vi "Main.vi"() -> (0 "error out":errorcluster)   [LabVIEW 2010, in "Sound Demo.lvclass"]
doc: "This is the top-level VI that starts the Sound Player Demo application."
uses:
  Sound Demo.lvclass
  Application/Application.lvclass
panel:
  # "This is the top-level VI of the \nSound Player Demo project."
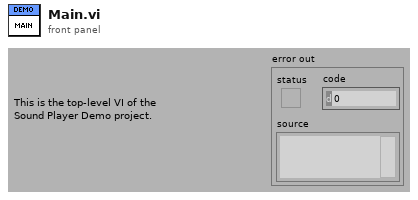
[diagram p1: front panel]
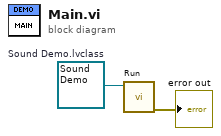
[diagram p0: block diagram]
diagram:
  w1 = refnum<class "Sound Demo.lvclass"> refnum  # Sound Demo.lvclass
  n1 = call "Run.vi"("Application in"=w1) -> ("error out"=→"error out":errorcluster)  [unwired: 9 in, 1 out]
